vi "Save Channel Groups to SoftCAL.vi"(0 "file path (dialog if empty)":path) -> (4 "file path out":path)   [LabVIEW 2019]
uses:
  Type Defs and Controls/Channel List.ctl
  Type Defs and Controls/Channel Config.ctl
  Type Defs and Controls/DAQ Settings.ctl
  Type Defs and Controls/Header.ctl
  Type Defs and Controls/Sensor Config.ctl
  Type Defs and Controls/Part Info.ctl
  Type Defs and Controls/All Part Info.ctl
  Type Defs and Controls/Test Limits.ctl
  Type Defs and Controls/Graph Settings Type Def.ctl
  Type Defs and Controls/Log File Type.ctl
  Type Defs and Controls/Trigger Stop Method.ctl
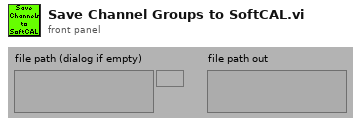
[diagram p1: front panel]
types:
  T1 = cluster{"Channel ID":string, "Channel Name":string, "Channel Type":enum16{"Voltage", "Thermocouple"}, "Selected Sensor":string, "Alarm Config":cluster{"Action":enum16{"Disabled", "Display On-Screen Warning", "Shutdown System"}, "Low Limit":dbl, "High Limit":dbl}, "Thermocouple Info":cluster{"Thermocouple Type":u16, "Temperature Units":u16, "Temperature Low Limit":sgl, "Temperature High Limit":sgl, "CJC Sensor Type":u16, "Thermistor Excitation":u16, "CJC Channel ID":u16, "Dedicated CJTEMP for Channel":u16, "Use CALGND":u16, "Dedicated CALGND for Channel":u16}}
  T2 = typedef "Sensor Config.ctl" = cluster{"DAQ Settings":T3, "Channels":T6[], "Header":T7, "Graph Settings":T8, "Test Limits":T9[], "All Type Info":T10, "Save Mode":enum16{"Single File", "Segmented Files", "New File at Midnight"}}
  T3 = typedef "DAQ Settings.ctl" = cluster{"Trigger Type":enum16{"Manual", "Timed", "Analog Rising", "Analog Falling"}, "Trigger Samples":i32, "Pretrigger Samples":i32, "Trigger Interval":dbl, "Time Units":bool, "Auto Save":bool, "Sample Rate":dbl, "Select Analog":bool, "Trigger Value":dbl, "Trigger Stop Method":T4, "Rate Sec/Min":bool, "Save Mode":enum16{"Single File", "Segmented Files", "New File at Midnight"}, "File Size Limit":dbl, "Log File Type":T5, "Trigger Data Index":u32}
  T4 = typedef "Trigger Stop Method.ctl" = enum16{"Use Samples Value to Stop Trigger", "Use Threshold to Stop Trigger"}
  T5 = typedef "Log File Type.ctl" = enum16{"Basic", "RTS"}
  T6 = typedef "Channel Config.ctl" = cluster{"Channel":string, "Type":string, "Acquire":bool, "Name":string, "Sensor":string, "Data Index":u32}
  T7 = typedef "Header.ctl" = cluster{"TA Number":string, "Test Name":string, "Serial Number":string, "Technician":string}
  T8 = typedef "Graph Settings Type Def.ctl" = cluster{"Graph Labels":string[], u8[], i16[], u32[], u8[], u8[], u8[], u32[], u8[], u8[], u8[], dbl[], dbl[], "Graph Toggles":bool[], "Axis Toggles":bool[], "Graph Range":enum16{"1", "2", "3", "4", "5", "10", "15", "30", "60"}}
  T9 = typedef "Test Limits.ctl" = cluster{"Channel Acquired?":bool, "RMS?":bool, "Pk-Pk":bool, "Frequency":bool, "EU High Limit 1":dbl, "EU Low Limit 1":dbl, "EU High Limit 2":dbl, "EU Low Limit 2":dbl, "RMS High Limit":dbl, "RMS Low Limit":dbl, "Pk-Pk High Limit ":dbl, "Pk-Pk Low Limit":dbl, "Frequency High Limit":dbl, "Frequency Low Limit":dbl}
  T10 = typedef "All Part Info.ctl" = cluster{"Type Name":string, "Type Signal Names":string[], "# Signals":i32, "# Parts":i32, "Part Info":T11[]}[]
  T11 = typedef "Part Info.ctl" = cluster{"Part Number":string, "Channel Indexes":u16[], "Enabled?":bool}
  T12 = typedef "Channel List.ctl" = cluster{"Device":i16, "Channels":cluster{"Channel ID":string, "Channel Name":string, "Channel Type":enum16{"Voltage", "Thermocouple"}, "Selected Sensor":string, "Alarm Config":cluster{"Action":enum16{"Disabled", "Display On-Screen Warning", "Shutdown System"}, "Low Limit":dbl, "High Limit":dbl}, "Thermocouple Info":cluster{"Thermocouple Type":u16, "Temperature Units":u16, "Temperature Low Limit":sgl, "Temperature High Limit":sgl, "CJC Sensor Type":u16, "Thermistor Excitation":u16, "CJC Channel ID":u16, "Dedicated CJTEMP for Channel":u16, "Use CALGND":u16, "Dedicated CALGND for Channel":u16}}[]}[]
  T13 = enum16{"Manual", "Timed", "Analog Rising", "Analog Falling"}
  T14 = cluster{"Channel ID":string, "Channel Name":string, "Channel Type":enum16{"Voltage", "Thermocouple"}, "Selected Sensor":string, "Alarm Config":cluster{"Action":enum16{"Disabled", "Display On-Screen Warning", "Shutdown System"}, "Low Limit":dbl, "High Limit":dbl}, "Thermocouple Info":cluster{"Thermocouple Type":u16, "Temperature Units":u16, "Temperature Low Limit":sgl, "Temperature High Limit":sgl, "CJC Sensor Type":u16, "Thermistor Excitation":u16, "CJC Channel ID":u16, "Dedicated CJTEMP for Channel":u16, "Use CALGND":u16, "Dedicated CALGND for Channel":u16}}[]
  T15 = cluster{"Device":i16, "Channels":cluster{"Channel ID":string, "Channel Name":string, "Channel Type":enum16{"Voltage", "Thermocouple"}, "Selected Sensor":string, "Alarm Config":cluster{"Action":enum16{"Disabled", "Display On-Screen Warning", "Shutdown System"}, "Low Limit":dbl, "High Limit":dbl}, "Thermocouple Info":cluster{"Thermocouple Type":u16, "Temperature Units":u16, "Temperature Low Limit":sgl, "Temperature High Limit":sgl, "CJC Sensor Type":u16, "Thermistor Excitation":u16, "CJC Channel ID":u16, "Dedicated CJTEMP for Channel":u16, "Use CALGND":u16, "Dedicated CALGND for Channel":u16}}[]}
  T16 = cluster{"Device":i16, "Channels":cluster{"Channel ID":string, "Channel Name":string, "Channel Type":enum16{"Voltage", "Thermocouple"}, "Selected Sensor":string, "Alarm Config":cluster{"Action":enum16{"Disabled", "Display On-Screen Warning", "Shutdown System"}, "Low Limit":dbl, "High Limit":dbl}, "Thermocouple Info":cluster{"Thermocouple Type":u16, "Temperature Units":u16, "Temperature Low Limit":sgl, "Temperature High Limit":sgl, "CJC Sensor Type":u16, "Thermistor Excitation":u16, "CJC Channel ID":u16, "Dedicated CJTEMP for Channel":u16, "Use CALGND":u16, "Dedicated CALGND for Channel":u16}}[]}[]
  T17 = typedef "Registry refnum.ctl" = refnum<k1>
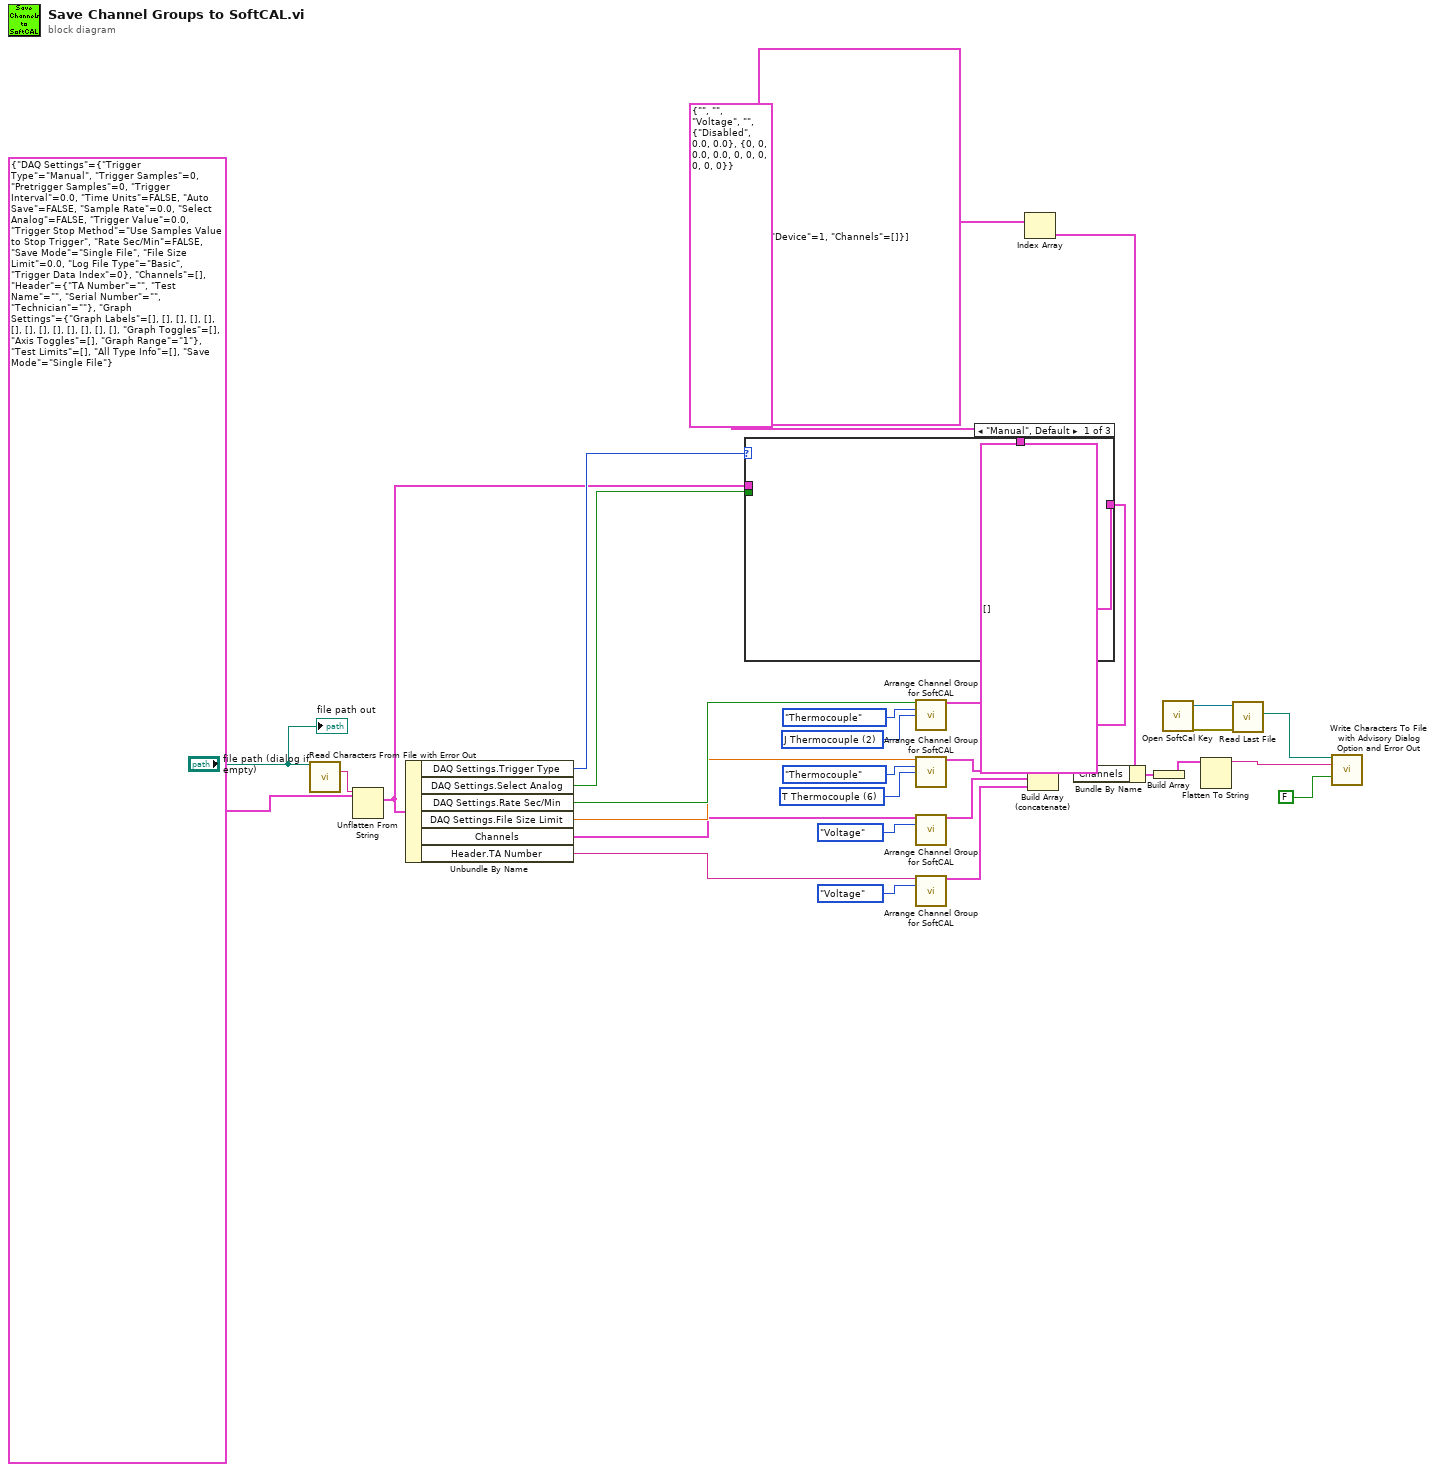
[diagram p0: block diagram]
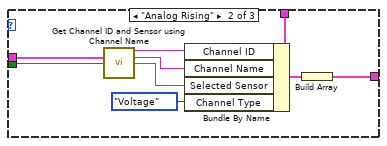
[diagram p2: hidden frame]
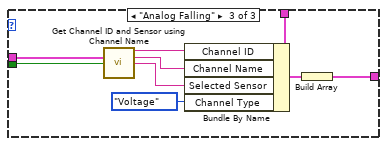
[diagram p3: hidden frame]
diagram:
  w27 = u16 6 items=["B Thermocouple", "E Thermocouple", "J Thermocouple", "K Thermocouple", "R Thermocouple", "S Thermocouple", "T Thermocouple", "N Thermocouple"] ("Thermocouple Type")
  w29 = u16 2 items=["B Thermocouple", "E Thermocouple", "J Thermocouple", "K Thermocouple", "R Thermocouple", "S Thermocouple", "T Thermocouple", "N Thermocouple"] ("Thermocouple Type")
  n1 = call "Read Characters From File with Error Out.vi"("file path (dialog if empty)"="file path (dialog if empty)") -> ("character string"=w32:string)  [unwired: 10 in, 4 out]
  n2 = Unflatten From String(type=T2 {"DAQ Settings"={"Trigger Type"=enum."Manual", "Trigger Samples"=0, "Pretrigger Samples"=0, "Trigger Interval"=0.0, "Time Units"=FALSE, "Auto Save"=FALSE, "Sample Rate"=0.0, "Select Analog"=FALSE, "Trigger Value"=0.0, "Trigger Stop Method"=enum."Use Samples Value to Stop Trigger", "Rate Sec/Min"=FALSE, "Save Mode"=enum."Single File", "File Size Limit"=0.0, "Log File Type"=enum."Basic", "Trigger Data Index"=0}, "Channels"=[], "Header"={"TA Number"="", "Test Name"="", "Serial Number"="", "Technician"=""}, "Graph Settings"={"Graph Labels"=[], [], [], [], [], [], [], [], [], [], [], [], [], "Graph Toggles"=[], "Axis Toggles"=[], "Graph Range"=enum."1"}, "Test Limits"=[], "All Type Info"=[], "Save Mode"=enum."Single File"} ("Config"), binary string=w32) -> (value=w2:T2)  [unwired: 3 in, 2 out]
  n3 = Unbundle By Name(w2) -> ("DAQ Settings.Trigger Type"=w5:T13, "DAQ Settings.Select Analog"=w3:bool, "DAQ Settings.Rate Sec/Min"=w28:bool, "DAQ Settings.File Size Limit"=w23:dbl, "Channels"=w22:T6[], "Header.TA Number"=w21:string)
  n4 = case shown="\"Manual\", Default" w5 {
    tunnel: T1 {"Channel ID"="", "Channel Name"="", "Channel Type"=enum."Voltage", "Selected Sensor"="", "Alarm Config"={"Action"=enum."Disabled", "Low Limit"=0.0, "High Limit"=0.0}, "Thermocouple Info"={"Thermocouple Type"=0, "Temperature Units"=0, "Temperature Low Limit"=0.0, "Temperature High Limit"=0.0, "CJC Sensor Type"=0, "Thermistor Excitation"=0, "CJC Channel ID"=0, "Dedicated CJTEMP for Channel"=0, "Use CALGND"=0, "Dedicated CALGND for Channel"=0}} ("Channel Config") -> [_ w42 w51]
    tunnel: w3 -> [_ w41 w50]
    tunnel: w2 -> [_ w40 w49]
    tunnel: [T14 [] w34 w43] -> w1
    frame "Manual", Default {
    }
    frame "Analog Rising" {
      n5 = call "Get Channel ID and Sensor using Channel Name.vi"("Config"=w40, "Channel Name"=w41) -> ("Channel ID"=w39:string, "Channel Name"=w38:string, "Sensor"=w37:string)  [unwired: 11 in]
      n6 = Bundle By Name(cluster=w42, "Channel ID"=w39, "Channel Name"=w38, "Selected Sensor"=w37, "Channel Type"=enum16{"Voltage", "Thermocouple"}."Voltage") -> (w35:T1)
      n7 = Build Array(w35) -> (w34:T14)
    }
    frame "Analog Falling" {
      n8 = call "Get Channel ID and Sensor using Channel Name.vi"("Config"=w49, "Channel Name"=w50) -> ("Channel ID"=w48:string, "Channel Name"=w47:string, "Sensor"=w46:string)  [unwired: 11 in]
      n9 = Bundle By Name(cluster=w51, "Channel ID"=w48, "Channel Name"=w47, "Selected Sensor"=w46, "Channel Type"=enum16{"Voltage", "Thermocouple"}."Voltage") -> (w44:T1)
      n10 = Build Array(w44) -> (w43:T14)
    }
  }
  n11 = call "Arrange Channel Group for SoftCAL.vi"("Channel Group"=w28, "Channel Type"=enum16{"Voltage", "Thermocouple"}."Thermocouple", "Thermocouple Type"=w29) -> ("SoftCAL Channel Config"=w20:T14)  [unwired: 12 in]
  n12 = call "Arrange Channel Group for SoftCAL.vi"("Channel Group"=w23, "Channel Type"=enum16{"Voltage", "Thermocouple"}."Thermocouple", "Thermocouple Type"=w27) -> ("SoftCAL Channel Config"=w19:T14)  [unwired: 12 in]
  n13 = call "Arrange Channel Group for SoftCAL.vi"("Channel Group"=w22, "Channel Type"=enum16{"Voltage", "Thermocouple"}."Voltage") -> ("SoftCAL Channel Config"=w18:T14)  [unwired: 13 in]
  n14 = call "Arrange Channel Group for SoftCAL.vi"("Channel Group"=w21, "Channel Type"=enum16{"Voltage", "Thermocouple"}."Voltage") -> ("SoftCAL Channel Config"=w17:T14)  [unwired: 13 in]
  n15 = Index Array(array=T12 [{"Device"=1, "Channels"=[]}] ("Configuration")) -> (element=w15:T15)  [unwired: 1 in]
  n16 = Build Array (concatenate)(w1, w20, w19, w18, w17) -> (w14:T14)
  n17 = Bundle By Name(cluster=w15, "Channels"=w14) -> (w13:T15)
  n18 = Build Array(w13) -> (w10:T16)
  n19 = call "Open SoftCal Key.vi"() -> ("error out"=w11:errorcluster, "refnum out"=w12:T17)  [unwired: 6 in]
  n20 = Flatten To String(anything=w10) -> (data string=w8:string)  [unwired: 3 in, 2 out]
  n21 = call "Read Last File.vi"("error in (no error)"=w11, "refnum"=w12) -> ("Last File"=w7:path)  [unwired: 3 in, 2 out]
  n22 = call "Write Characters To File with Advisory Dialog Option and Error Out.vi"("file path (dialog if empty)"=w7, "character string"=w8, "advisory dialog? (display:T)"=FALSE) -> ()  [unwired: 11 in, 2 out]
  "file path out" <- "file path (dialog if empty)"
